vi "VISA_WRITE.vi"(3 "error in (no error)":errorcluster, 4 "write buffer":string, 5 "VISA resource name":refnum<visa-resource-name>) -> (0 "error out":errorcluster, 1 "return count":u32, 2 "dup VISA resource name":refnum<visa-resource-name>)   [LabVIEW 2012]
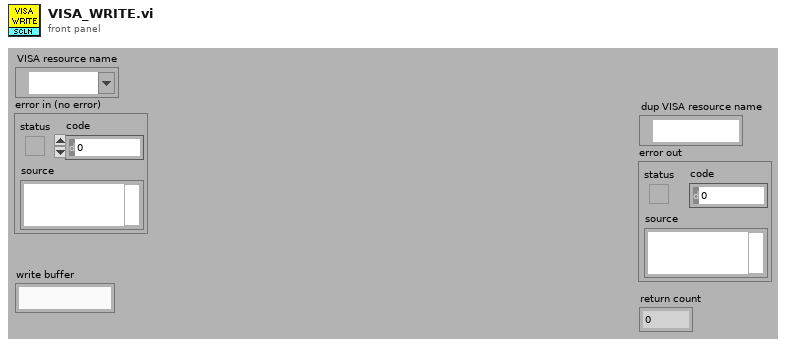
[diagram p1: front panel]
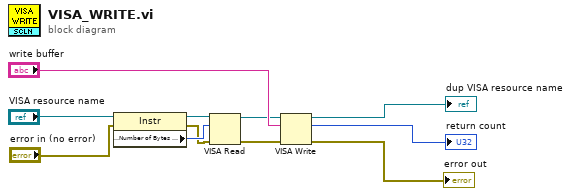
[diagram p0: block diagram]
diagram:
  n1 = property class="Instr"(reference="VISA resource name", error in="error in (no error)") -> (reference out=w7:refnum<visa-resource-name>, error out=w5:errorcluster, "Serial Settings:Number of Bytes at Serial Port"=w6:u32)
  n2 = VISA Read(VISA resource name=w7, byte count=w6, error in (no error)=w5) -> (VISA resource name out=w3:refnum<visa-resource-name>, error out=w4:errorcluster)  [unwired: 2 out]
  n3 = VISA Write(VISA resource name=w3, write buffer="write buffer", error in (no error)=w4) -> (VISA resource name out=→"dup VISA resource name":refnum<visa-resource-name>, return count=→"return count":u32, error out=→"error out":errorcluster)
